vi "user event out globals - SubVI.vi"() -> ()   [LabVIEW 2014]
uses:
  Glimpse-master/Microscope plugins/Stage/Move stage command.ctl
panel:
  out "user event out":refnum<user-event>
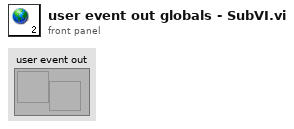
[diagram p1: front panel]
diagram:
